vi "CreateClass.vi"(7 "PythonConverter_BD in":refnum<class "PyConvBD.lvclass">, 8 "error in":errorcluster, 11 "Diagram in":refnum<class "Diagram.lvclass">) -> (0 "error out":errorcluster, 3 "Diagram out":refnum<class "Diagram.lvclass">, 4 "diagram":string, 5 "PythonConverter_BD out":refnum<class "PyConvBD.lvclass">)   [LabVIEW 2014, in "Raspberry Pi Compatible Compiler for LabVIEW.lvlib" / "Diagram.lvclass"]
uses:
  Diagram.lvclass
  Python/PythonConverter_BD/PyConvBD.lvclass
  Python/Parsing/ClassTypeTD.ctl
  Python/Parsing/Python Functions.lvlib
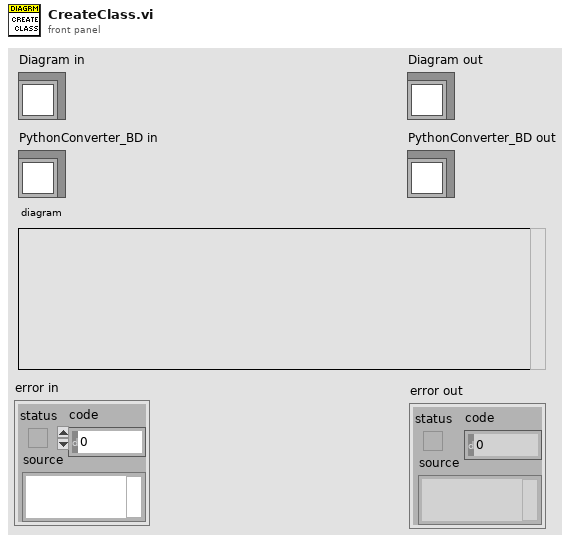
[diagram p1: front panel]
types:
  T1 = typedef "Raspberry Pi Compatible Compiler for LabVIEW.lvlib/Python Functions.lvlib/ClassTypeTD.ctl" = enum16{"class", "function"}
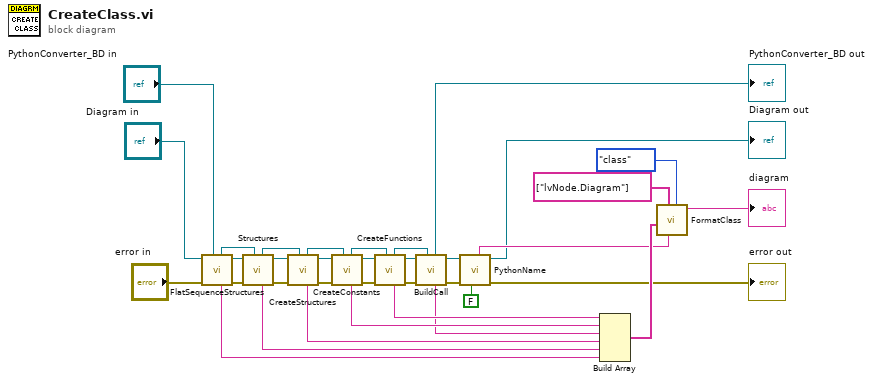
[diagram p0: block diagram]
diagram:
  n1 = call "FlatSequenceStructures.vi"("PythonConverter_BD in"="PythonConverter_BD in", "error in"="error in", "Diagram in"="Diagram in") -> ("error out"=w4:errorcluster, "Diagram out"=w7:refnum<class "Diagram.lvclass">, "fss"=w1:string, "PythonConverter_BD out"=w6:refnum<class "PyConvBD.lvclass">)  [unwired: 5 in]
  n2 = call "Structures.vi"("PythonConverter_BD in"=w6, "error in"=w4, "Diagram in"=w7) -> ("error out"=w10:errorcluster, "Diagram out"=w11:refnum<class "Diagram.lvclass">, "structures"=w2:string, "PythonConverter_BD out"=w9:refnum<class "PyConvBD.lvclass">)  [unwired: 5 in]
  n3 = call "CreateStructures.vi"("PythonConverter_BD in"=w9, "error in"=w10, "Diagram in"=w11) -> ("error out"=w29:errorcluster, "Diagram out"=w28:refnum<class "Diagram.lvclass">, "create structures"=w19:string, "PythonConverter_BD out"=w27:refnum<class "PyConvBD.lvclass">)  [unwired: 5 in]
  n4 = call "CreateConstants.vi"("PythonConverter_BD in"=w27, "error in"=w29, "Diagram in"=w28) -> ("error out"=w34:errorcluster, "Diagram out"=w35:refnum<class "Diagram.lvclass">, "create constants"=w21:string, "PythonConverter_BD out"=w26:refnum<class "PyConvBD.lvclass">)  [unwired: 5 in]
  n5 = call "CreateFunctions.vi"("PythonConverter_BD in"=w26, "error in"=w34, "Diagram in"=w35) -> ("error out"=w33:errorcluster, "Diagram out"=w31:refnum<class "Diagram.lvclass">, "create functions"=w22:string, "PythonConverter_BD out"=w32:refnum<class "PyConvBD.lvclass">)  [unwired: 5 in]
  n6 = call-dynamic "BuildCall.vi"("PythonConverter_BD in"=w32, "error in"=w33, "Diagram in"=w31) -> ("error out"=w16:errorcluster, "Diagram out"=w17:refnum<class "Diagram.lvclass">, "diagram"=w20:string, "PythonConverter_BD out"=→"PythonConverter_BD out":refnum<class "PyConvBD.lvclass">)  [unwired: 5 in]
  n7 = call-dynamic "PythonName.vi"("add self"=FALSE, "error in"=w16, "Diagram in"=w17) -> ("error out"=→"error out":errorcluster, "Diagram out"=→"Diagram out":refnum<class "Diagram.lvclass">, "name"=w15:string)  [unwired: 5 in, 1 out]
  n8 = Build Array(w22, w21, w20, w19, w2, w1) -> (w18:string[])
  n9 = call "FormatClass.vi"("type"=ClassTypeTD."class", "name"=w15, "parameters/ancestors"=string[] ["lvNode.Diagram"], "body"=w18) -> ("python"=→"diagram":string)  [unwired: 7 in]
